vi "put_chair_cushions.vi"(8 "error in":errorcluster, 11 "chairs in":refnum<class "Chair.lvclass">[](array[class])) -> (0 "error out":errorcluster, 2 "results":string[](array[string]), 3 "chairs in 2":refnum<class "Chair.lvclass">[](array[class]))   [LabVIEW 2021]
uses:
  Chair.lvclass
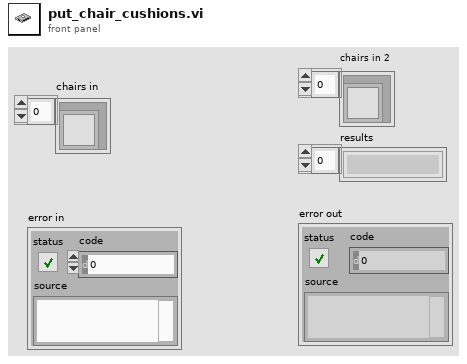
[diagram p1: front panel]
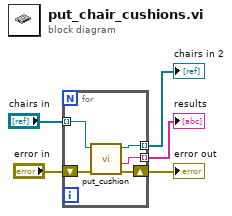
[diagram p0: block diagram]
diagram:
  n1 = for {
    tunnel: "chairs in" -> [w10] mode=indexing
    tunnel: [w9] -> w4 mode=indexing
    tunnel: [w8] -> w3 mode=indexing
    shift-right: [w6] -> w1
    shift-left: "error in" -> [w7]
    n2 = call-dynamic "put_cushion.vi"("error in (no error)"=w7, "Chair in"=w10) -> ("error out"=w6:errorcluster, "result"=w8:string, "Chair out"=w9:refnum<class "Chair.lvclass">)  [unwired: 7 in]
  }
  "chairs in 2" <- w4
  "results" <- w3
  "error out" <- w1
